vi "FLiBe Viscosity.vi"(11 "Temperature (K)":dbl) -> (3 "FLiBe Viscosity (Pa-s)":dbl)   [LabVIEW 2019]
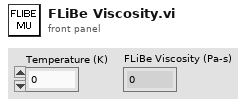
[diagram p1: front panel]
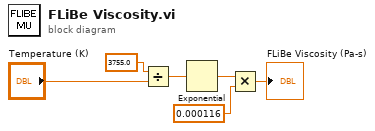
[diagram p0: block diagram]
diagram:
  n1 = Divide(x=3755.0, y="Temperature (K)") -> (x/y=w2:dbl)
  n2 = Exponential(1:w2) -> (0:w5:dbl)
  n3 = Multiply(x=w5, y=0.000116) -> (x*y=→"FLiBe Viscosity (Pa-s)":dbl)
